vi "SET_G_EQUIP_COMM.vi"(10 "conn status":bool, 11 "interface name":string) -> ()   [LabVIEW 2018]
uses:
  G_EQUIP_CMM.vi
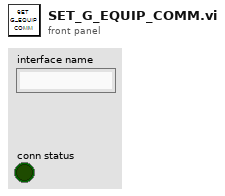
[diagram p1: front panel]
types:
  T1 = typedef "Semaphore RefNum" = refnum<k1>
  T2 = cluster{"P/S":bool, "A-CAN1":bool, "A-CAN2":bool, "D-CAN":bool, "R-CAN":bool, "E-CAN":bool, "AIO-6229":bool, "DIO-6229":bool, "DAQ-7432":bool, "DMM":bool}
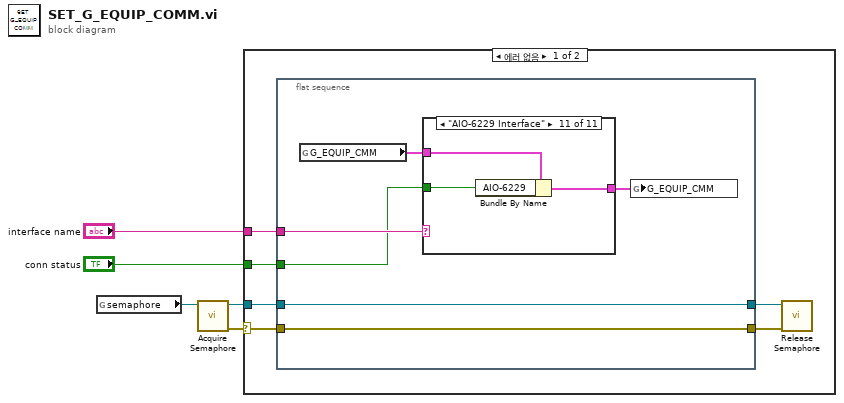
[diagram p0: block diagram]
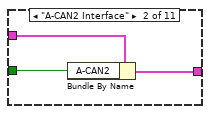
[diagram p3: hidden frame]
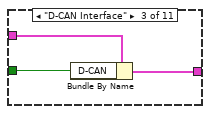
[diagram p4: hidden frame]
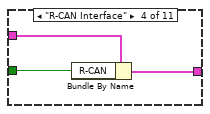
[diagram p5: hidden frame]
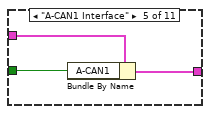
[diagram p6: hidden frame]
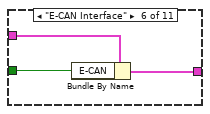
[diagram p7: hidden frame]
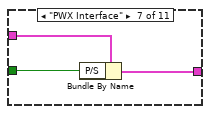
[diagram p8: hidden frame]
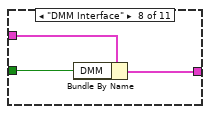
[diagram p9: hidden frame]
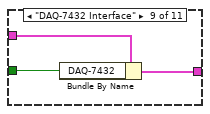
[diagram p10: hidden frame]
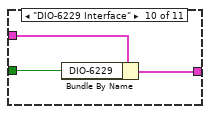
[diagram p11: hidden frame]
diagram:
  n1 = global read "G_EQUIP_CMM.vi" "semaphore"() -> (w3:T1)
  n2 = call <vilib>:"Acquire Semaphore.vi"("semaphore"=w3) -> ("error out"=w2:errorcluster, "semaphore out"=w1:T1)  [unwired: 4 in, 1 out]
  n3 = case shown="에러 없음" w2 {
    selector: w2 -> [w8 _]
    tunnel: "interface name" -> [w11 _]
    tunnel: "conn status" -> [w10 _]
    tunnel: w1 -> [w9 _]
    frame No Error {
      n4 = flat-sequence {
        tunnel: w11 -> [w15]
        tunnel: w10 -> [w14]
        tunnel: w9 -> [w13]
        tunnel: w8 -> [w12]
        tunnel: [w13] -> w7
        tunnel: [w12] -> w6
        frame #0 {
          n5 = global read "G_EQUIP_CMM.vi" "G_EQUIP_CMM"() -> (w16:T2)
          n6 = case shown="\"AIO-6229 Interface\"" w15 {
            tunnel: w16 -> [w18 w21 w24 w27 w30 w33 w36 w39 w42 w45 w48]
            tunnel: [w18 w20 w23 w26 w29 w31 w34 w37 w40 w43 w46] -> w17
            tunnel: w14 -> [_ w19 w22 w25 w28 w32 w35 w38 w41 w44 w47]
            frame Default {
            }
            frame "A-CAN2 Interface" {
              n7 = Bundle By Name(cluster=w21, "A-CAN2"=w19) -> (w20:T2)
            }
            frame "D-CAN Interface" {
              n8 = Bundle By Name(cluster=w24, "D-CAN"=w22) -> (w23:T2)
            }
            frame "R-CAN Interface" {
              n9 = Bundle By Name(cluster=w27, "R-CAN"=w25) -> (w26:T2)
            }
            frame "A-CAN1 Interface" {
              n10 = Bundle By Name(cluster=w30, "A-CAN1"=w28) -> (w29:T2)
            }
            frame "E-CAN Interface" {
              n11 = Bundle By Name(cluster=w33, "E-CAN"=w32) -> (w31:T2)
            }
            frame "PWX Interface" {
              n12 = Bundle By Name(cluster=w36, "P/S"=w35) -> (w34:T2)
            }
            frame "DMM Interface" {
              n13 = Bundle By Name(cluster=w39, "DMM"=w38) -> (w37:T2)
            }
            frame "DAQ-7432 Interface" {
              n14 = Bundle By Name(cluster=w42, "DAQ-7432"=w41) -> (w40:T2)
            }
            frame "DIO-6229 Interface" {
              n15 = Bundle By Name(cluster=w45, "DIO-6229"=w44) -> (w43:T2)
            }
            frame "AIO-6229 Interface" {
              n16 = Bundle By Name(cluster=w48, "AIO-6229"=w47) -> (w46:T2)
            }
          }
          n17 = global write "G_EQUIP_CMM.vi" "G_EQUIP_CMM"(w17) -> ()
        }
      }
      n18 = call <vilib>:"Release Semaphore.vi"("error in (no error)"=w6, "semaphore"=w7) -> ()  [unwired: 4 in, 2 out]
    }
    frame Error {
    }
  }
